vi "DAQ Close.vi"(1 "error in":errorcluster, 2 "task in":refnum<k21>) -> (0 "error out":errorcluster)   [LabVIEW 2023]
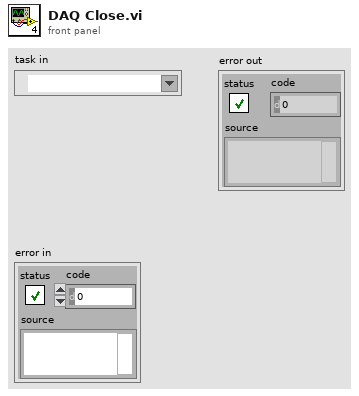
[diagram p1: front panel]
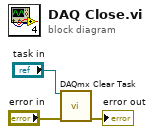
[diagram p0: block diagram]
diagram:
  n1 = call <vilib>:"DAQmx Clear Task.vi"("task in"="task in", "error in"="error in") -> ("error out"=→"error out":errorcluster)  [unwired: 13 in]
